vi "Max_Min_conversion.vi"(10 "Min":dbl, 11 "Max":dbl) -> (2 "offset":dbl, 3 "Amplitude":dbl)   [LabVIEW 2013]
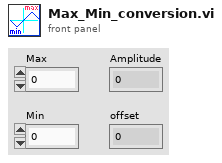
[diagram p1: front panel]
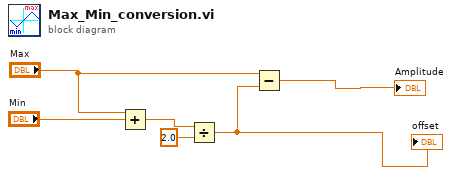
[diagram p0: block diagram]
diagram:
  n1 = Add(x="Max", y="Min") -> (x+y=w3:dbl)
  n2 = Divide(x=w3, y=2.0) -> (x/y=w5:dbl)
  "offset" <- w5
  n3 = Subtract(x="Max", y=w5) -> (x-y=→"Amplitude":dbl)
